vi "Main.vi"(7 "sweep rate, /min":dbl=0.2, 8 "sweep to:":dbl=-0.5, 9 "sweep":T6(radio)=enum."time_sweep") -> ()   [LabVIEW 2017]
uses:
  controls/Channel.ctl
  <instrlib>/Zurich Instruments LabOne/Public/ziTypeHandle.ctl
  controls/Measure.ctl
  controls/iPSreadCtrl.ctl
  controls/iTCreadCtrl.ctl
  subVIs/MFLIcommand.ctl
  controls/iPSsetCtrl.ctl
  controls/Source.ctl
  controls/iTCsetCtrl.ctl
  <vilib>/Utility/file.llb/Write To Spreadsheet File (DBL).vi
  <vilib>/gmath/NI_Gmath.lvlib
  <instrlib>/Keithley 2450/Keithley 2450.lvlib
  HULK SMS/SMScontrols.ctl
  <instrlib>/Zurich Instruments LabOne/Zurich Instruments LabOne.lvlib
panel:
  in  "Lead Chanl":T1(ring)=enum."time_sweep"
  in  "Sweep Up":bool
  in  "Stop Ramp":bool
  in  "Up Rate":dbl
  in  "Down Rate":dbl
  in  "Ramp \nUp":bool
  in  "Ramp\n Down":bool
  in  "lower limit":dbl=-4.0
  in  "upper limit":dbl=4.0
  in  "Sweep Down":bool
  in  "Stop Sweep":bool
  in  "Continuous Sweep":bool
  in  "Slave Chanl":T2=enum."b"
  in  "Double Sweep":bool
  in  "Slope":dbl
  in  "Offset":dbl
  in  "time/point, sec":dbl=2.0
  out "sweep value":dbl=2.186666666666735
  out "time delay, ms":dbl
  out "current time":timestamp=timestamp(3589630313.018 s since 1904-01-01) format="%<%H:%M:%S%1u>T"
  in  "Step and Hyerloop Setups":T3(tab)
  in  "Tab Control":T4(tab)
  in  "MFLI_I2":bool
  in  "MFLI_V2":bool
  in  "MFLI_2":string="DEV5142"
  in  "SR830_8_oop":bool
  in  "SR830_7_oop":bool
  in  "SR830_8_ip":bool
  in  "SR830_7_ip":bool
  in  "SR830_6_oop":bool
  in  "SR830_6_ip":bool
  in  "SR830_8":u8=8
  in  "SR830_7":u8=7
  in  "SR830_6":u8=6
  in  "MFLI_I1":bool
  in  "MFLI_V1":bool
  in  "MFLI_1":string="DEV5150"
  in  "SR830 5 oop":bool
  in  "SR830 5 ip":bool
  in  "SR830 5 addr":u8=5
  in  "SR830 4 oop":bool
  in  "SR830 4 ip":bool
  in  "SR830 3 oop":bool
  in  "SR830 3 ip":bool
  in  "SR830 2 oop":bool
  in  "SR830 2 ip":bool
  in  "SR830 1 oop":bool
  in  "SR830 1 ip":bool
  in  "SR830 4 addr":u8=4
  in  "SR830 3 addr":u8=3
  in  "SR830 2 addr":u8=2
  in  "SR830 1 addr":u8=1
  in  "VTI_P":bool
  in  "PT2_T":bool
  in  "VTI_T":bool
  in  "PT1_T":bool
  in  "SH_T":bool
  in  "Magnet_T":bool
  in  "2182A 4 ch2":bool
  in  "2182A 4 ch1":bool
  in  "2182A 3 ch2":bool
  in  "2182A 3 ch1":bool
  in  "2182A 2 ch2":bool
  in  "2182A 2 ch1":bool
  in  "2182A 4 addr":u8=18
  in  "2182A 3 addr":u8=17
  in  "2182A 2 addr":u8=16
  in  "2182A 1 addr":u8=15
  in  "2182A 1 ch2":bool
  in  "2182A 1 ch1":bool
  out "HandleOut":T5 {"Handle" format="0x%08x"; "Conn" format="0x%08x"}
  out "Handle Out 2":T5 {"Handle" format="0x%08x"; "Conn" format="0x%08x"}
  in  "Step Loop":bool
  in  "Sweep B":bool
  in  "2461_addr_sweep":refnum<visa-resource-name>="itcetherT"
  in  "2461_meas_i":bool
  in  "2461_meas_v":bool
  in  "Tolerance_Sweep":dbl=0.01
  in  "iTC_Sample_T":bool
  in  "iTC_addr_sweep":refnum<visa-resource-name>="iTC"
  in  "iPS_addr_sweep":refnum<visa-resource-name>="iPS"
  in  "2400 3 addr":u8=14
  in  "2400 2 addr":u8=12
  in  "2400 1 addr":u8=13
  in  "2336A addr":refnum<visa-resource-name>="Keithley2614B"
  in  "sweep 2":bool
  in  "iPS_MagnetField":bool
  in  "auto\nrange B":bool
  in  "measure time":bool
  in  "2636A smub meas i":bool
  in  "2636A smub meas v":bool
  in  "2636A smua meas i":bool
  in  "2636A smua meas v":bool
  in  "2400 3 meas i":bool
  in  "2400 2 meas i":bool
  in  "2400 2 meas v":bool
  in  "2400 3 meas v":bool
  in  "2400 1 meas i":bool
  in  "2400 1 meas v":bool
  in  "auto\nrange A":bool
  in  "SlaveUpLimit":dbl
  in  "SlaveDownLimit":dbl
  in  "Change Doule Sweep OffSet":bool
  in  "Lead Chanl_step":T7(ring)=enum."2636a_smua_step" caption="Lead Chanl"
  in  "UpLimitValue":dbl
  in  "DownLimitValue":dbl
  in  "Change Sweep Range":bool
  in  "Offset_Up":dbl
  in  "Offset_Down":dbl
  in  "Slope":dbl
  in  "Down          Up":string[][](table)
  in  "Generate":bool
  in  "2461_addr_step":refnum<visa-resource-name>="itcetherT"
  in  "Channel":T2=enum."b"
  in  "Mini steps":dbl=30.0
  in  "Tolerance_Step":dbl=0.01
  in  "Step Slope":dbl
  in  "Step Offset":dbl
  in  "diagonal step":bool
  in  "FieldRate(T/min)":dbl=0.1
  out "at field":bool
  in  "iPS _addr_step":refnum<visa-resource-name>="iPS"
  in  "iTC_addr_step":refnum<visa-resource-name>="iTC"
  in  "step":T8(radio)=enum."time_step"
  in  "2336A_addr_step":refnum<visa-resource-name>="Keithley2614B"
  in  "2400_2_addr_step":u8=12
  in  "2400_1_addr_step":u8=12
  in  "wait between sweeps(s)":u32=1
  in  "Wait Between Step(s)":i32=1
  in  "Stop Mapping":bool
  in  "Start Mapping":bool
  in  "HyperLoop":bool
  in  "EstimateTime":bool
  out "MM:":dbl
  out "SS:":dbl
  out "HH:":dbl
  out "Finish Time":timestamp
  out "Sweep Direction":string
  out "Current Step Value":dbl
  out "Table Index":dbl
  in  "Populate step table?":bool
  in  "Step values":string[][](table)=[["-20"], ["-10"], ["-4"], ["-1"], ["3"], ["6"], ["10"], [""]]
  in  "to":dbl=1.0
  in  "step":dbl=2.0
  in  "from":dbl=1.0
  in  "SwapStepDirection":bool
  out "Hidden_HyperLoop_Swap":bool
  out "HyperLoop Hidden":bool
  in  "EstimateTime Hyper":bool
  out "MM:":dbl
  out "SS:":dbl
  out "HH:":dbl
  out "Finish Time 2":timestamp
  out "Sweep Direction 2":string
  out "Current Hyper Value":dbl
  out "HyperLoop Index":dbl
  in  "Populate HyperLoop table?":bool
  in  "HyperLoop Steps":string[][](table)=[["-20"], ["-10"], ["-4"], ["-1"], ["3"], ["6"], ["10"], [""]]
  in  "to":dbl=1.0
  in  "step":dbl=2.0
  in  "from":dbl=1.0
  in  "SuperHyper":bool
  in  "Channel_hyper":T2=enum."b"
  in  "Hyper_Mini steps":dbl=30.0
  in  "Tolerance_Hyper":dbl=0.1
  in  "Hyper Slope":dbl
  in  "Hyper Offset":dbl
  in  "diagonal_hyper":bool
  in  "Hyper_FieldRate\n(T/min)":dbl=0.1
  out "at field_hyper":bool
  in  "iPS _addr_hyper":refnum<visa-resource-name>="iPS"
  in  "iTC_addr_hyper":refnum<visa-resource-name>="iTC"
  in  "step_hyper":T9(radio)=enum."time_HyperLoop"
  in  "2336A_addr_hyper":refnum<visa-resource-name>="Keithley2614B"
  in  "2400_2_addr_hyper":u8=12
  in  "2400_1_addr_hyper":u8=12
  in  "Wait Between Hyper":i32=10
  in  "Stop HyperLoop":bool
  in  "Start HyperLoop":bool
  in  "SwapHyperDirection":bool
  out "Hidden_super_Swap":bool
  out "Super Hidden":bool
  in  "EstimateTime Hyper 2":bool
  out "MM:":dbl
  out "SS:":dbl
  out "HH:":dbl
  out "Finish Time Super":timestamp
  out "Sweep Direction3":string
  out "Current SuperHyper Value":dbl
  out "SuperHyper_Index":dbl
  in  "Populate SuperHyper table?":bool
  in  "SuperHyper Steps":string[][](table)=[["-20"], ["-10"], ["-4"], ["-1"], ["3"], ["6"], ["10"], [""]]
  in  "to":dbl=1.0
  in  "step":dbl=2.0
  in  "from":dbl=1.0
  in  "Channel_super":T2=enum."b"
  in  "Super_ministeps":dbl=30.0
  in  "Tolerance_super":dbl=0.1
  in  "Slope_super":dbl
  in  "Offset_super":dbl
  in  "diagona_super":bool
  in  "Super_FieldRate\n(T/min)":dbl=0.1
  out "at field_super":bool
  in  "iPS _addr_superhyper":refnum<visa-resource-name>="iPS"
  in  "iTC_addr_super":refnum<visa-resource-name>="iTC"
  in  "step_super":T10(radio)=enum."time_SuperHyper"
  in  "2336A_addr_super":refnum<visa-resource-name>="Keithley2614B"
  in  "2400_2_addr_super":u8=12
  in  "2400_1_addr_super":u8=12
  in  "Wait Btwn SuperHyper":i32=10
  in  "Stop SuperHyper":bool
  in  "StartSuperHyper":bool
  out "SuperHyper":dbl=-0.4901
  out "Hyper Channel":dbl=-0.4901
  out "Sweep Channel":dbl
  out "Step Channel":dbl=-0.4901
  in  "MappingName":string
  in  "Data Folder":path=path "F:/users/Yanmeng/Data"
  out "Data file:":path=path "D:/Yanmeng/Data/Year2018/January2018/Jan2318/Jan2318x001.dat"
  in  "Initialize":bool
  in  "Quit":bool
  in  "Refresh Time(ms)":u32=100
  in  "Monitor":bool
  out "DownNameString":string
  out "UpNameString":string
  in  "Cytec_Switch":bool
  in  "Lockin_Setup":bool
  in  "TempCtrl":bool
  in  "MagnetCtrl":bool
  out "status 3":bool
  in  "Y_right_formula":string="brty/10/(300*10^-9)"
  in  "Yright":u16(ring)=3 caption="Y-Right:" items=["V_sweep_2636a_smub", "SR830_1_ip", "SR830_1_oop", "SR830_2_ip", "SR830_2_oop", "SR830_3_ip", "SR830_3_oop", "SR830_4_ip", "SR830_4_oop", "2636A_smua_v", "2636A_smua_i", "2636A_smub_v", "2636A_smub_i", "iPS_MagntField", "iPS_Magnet_T", "iPS_SH_T", "iTC_Sample_T", "iTC_VTI_T", "iTC_PT1_T", "iTC_PT2_T", "iTC_VTI_P", "formula"]
  out "status 2":bool
  in  "Y_left_formula":string="brty/10/(300*10^-9)"
  in  "X_axis_formula":string
  in  "Yaxis":u16(ring)=3 caption="Y-Left:" items=["V_sweep_2636a_smub", "SR830_1_ip", "SR830_1_oop", "SR830_2_ip", "SR830_2_oop", "SR830_3_ip", "SR830_3_oop", "SR830_4_ip", "SR830_4_oop", "2636A_smua_v", "2636A_smua_i", "2636A_smub_v", "2636A_smub_i", "iPS_MagntField", "iPS_Magnet_T", "iPS_SH_T", "iTC_Sample_T", "iTC_VTI_T", "iTC_PT1_T", "iTC_PT2_T", "iTC_VTI_P", "formula"]
  out "XY Graph":cluster{"Y Values":dbl[], "Y Values":dbl[]}[](graph)
  in  "Xaxis":u16(ring) caption="X-axis:" items=["V_sweep_2636a_smub", "SR830_1_ip", "SR830_1_oop", "SR830_2_ip", "SR830_2_oop", "SR830_3_ip", "SR830_3_oop", "SR830_4_ip", "SR830_4_oop", "2636A_smua_v", "2636A_smua_i", "2636A_smub_v", "2636A_smub_i", "iPS_MagntField", "iPS_Magnet_T", "iPS_SH_T", "iTC_Sample_T", "iTC_VTI_T", "iTC_PT1_T", "iTC_PT2_T", "iTC_VTI_P", "formula"]
  out "status":bool
  in  "Show cursor":bool
  in  "Hulk_B_meas (Vnano)":bool
  in  "Hulk_SMS_addr":refnum<visa-resource-name>="TCPIP0::10.99.75.17::inst0::INSTR"
  in  "formula_variables":string[](array[string])=["a", "b", "c", "d", "e", "e", "f", "g", "h", "i", "j"]
  out "data":dbl[](array[numeric])
  out "Figure_axis":string[](array[string])=["HULK_SMS_output", "SR830_1_ip", "SR830_1_oop"]
  out "data_caption":string="HULK_SMS_output\tSR830_1_ip\tSR830_1_oop\t"
  # "Sweep Parameters Setup"
  # "Down"
  # "Up"
  # "Limits"
  # "Rate\n(/min)"
  # "Sweep Channel Setup"
  # "SweepChannel"
  # "address"
  # "sweep"
  # "2400_2"
  # "2400_3"
  # "2636A_smua"
  # "2636A_smub"
  # "time"
  # "Teslatron iPS"
  # "Teslatron iTC"
  # "2400_1"
  # "!Current sweep!"
  # "measure"
  # "Sample_T"
  # "MagnetField"
  # "voltage (_v)"
  # "current (_i)"
  # "Vtg"
  # "Vbg"
  # "Measure Channels"
  # "Lock-in amplifiers"
  # "address"
  # "SR830_1"
  # "SR830_2"
  # "SR830_3"
  # "SR830_4"
  # "measure"
  # "SR830_5"
  # "in phase (_ip)"
  # "out of phase (_oop)"
  # "Nanovoltmeters"
  # "Magnet&Temp"
  # "address"
  # "Equipment"
  # "iPS"
  # "iTC"
  # "measure"
  # "2182A_1"
  # "2182A_2"
  # "2182A_3"
  # "2182A_4"
  # "channel 1 (_ch1)"
  # "channel 2 (_ch2)"
  # "(not recommended, slow)"
  # "Step Channel Setup"
  # "StepChannel"
  # "addres"
  # "time"
  # "2400_1"
  # "2400_2"
  # "2636A_smua"
  # "2636A_smub"
  # "Teslatron iPS"
  # "Teslatron iTC"
  # "2461"
  # "step"
  # "Step Table"
  # "Step Table"
  # "Hyper Loop Setup"
  # "StepChannel"
  # "addres"
  # "Teslatron iPS"
  # "Teslatron iTC"
  # "2400_1"
  # "2400_2"
  # "2636A_smua"
  # "2636A_smub"
  # "time"
  # "step"
  # "SuperHyper Setup"
  # "StepChannel"
  # "addres"
  # "2400_1"
  # "2400_2"
  # "2636A_smua"
  # "2636A_smub"
  # "time"
  # "Teslatron iPS"
  # "Teslatron iTC"
  # "step"
  # "Step Table"
  # "Current Value of Sweep and Step Channels"
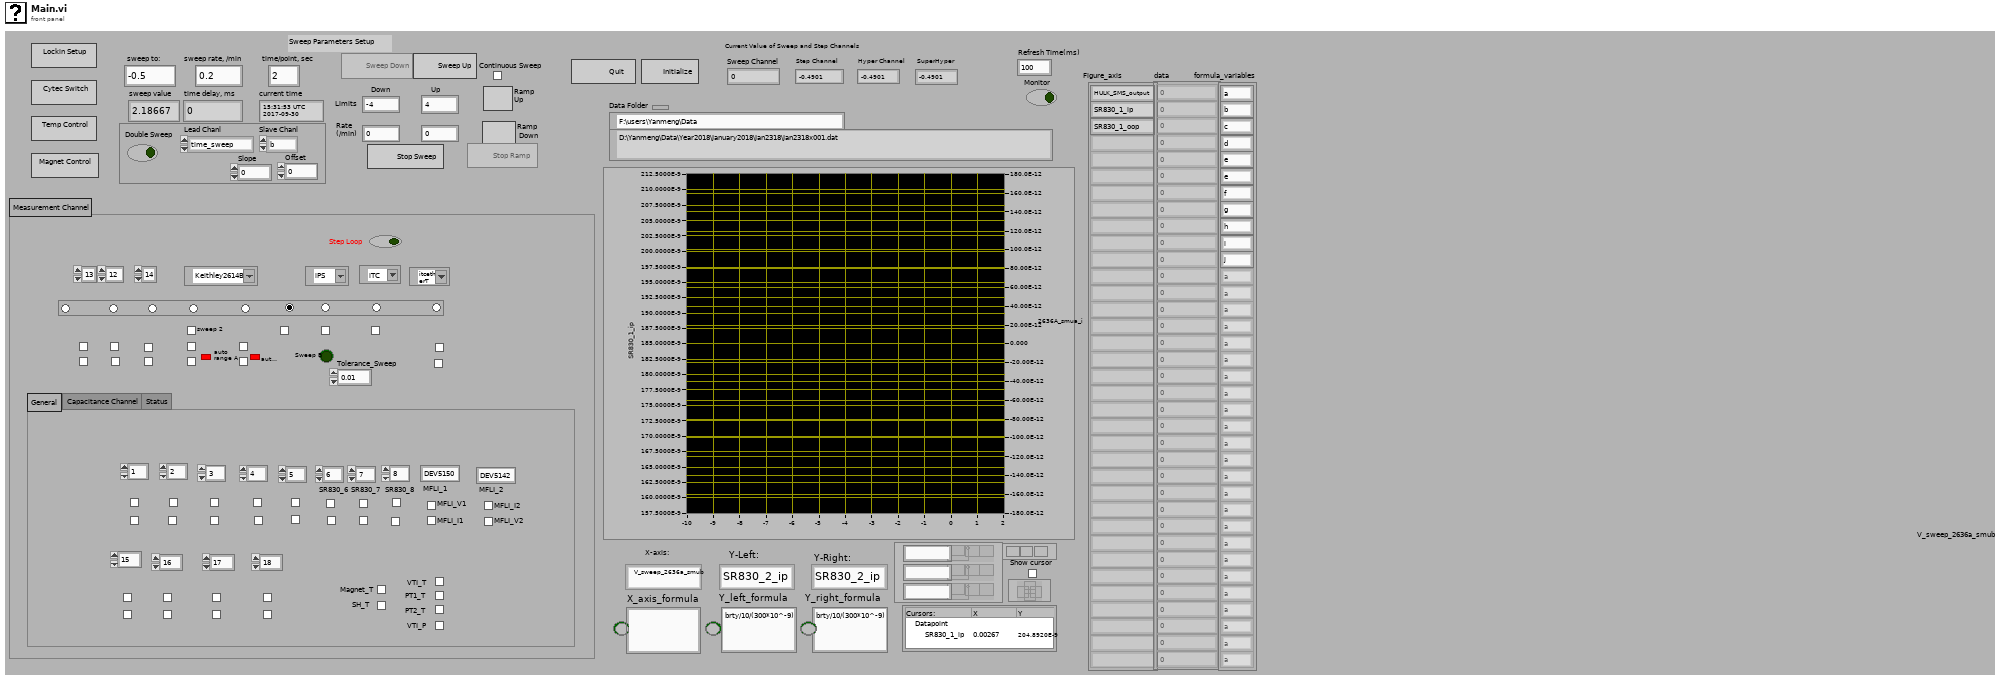
[diagram p1: front panel]
types:
  T1 = enum16{"2400_1", "2400_2", "2400_3", "2636a_smua", "2636a_smub", "time_sweep", "iPS", "iTC", "2461"}
  T2 = typedef "Channel.ctl" = enum16{"a", "b"}
  T3 = enum32{"Measurement Channel", "Step", "HyperLoop", "SuperHyper"}
  T4 = enum32{"General", "Capacitance Channel", "Status"}
  T5 = typedef "Zurich Instruments LabOne.lvlib/ziTypeHandle.ctl" = cluster{"handleValid":bool, "Conn":u64, "Path Prefix":string, "Handle":u64, "Connected":bool, "Clockbase(s)":dbl}
  T6 = enum32{"2400_1", "2400_2", "2400_3", "2636a_smua", "2636a_smub", "time_sweep", "iPS", "iTC", "2461"}
  T7 = enum16{"V2400_1_step", "V2400_2_step", "2636a_smua_step", "2636a_smub_step", "time_step", "iPS_step", "iTC_step", "2461_Curr"}
  T8 = enum32{"V2400_1_Step", "V2400_2_step", "2636_smua_step", "2636_smub_step", "time_step", "iTC_step", "iPS_step", "2461_Curr"}
  T9 = enum32{"2400_1_HyperLoop", "2400_2_HyperLoop", "2636_smua_HyperLoop", "2636_smub_HyperLoop", "time_HyperLoop", "iTC_HyperLoop", "iPS_HyperLoop"}
  T10 = enum32{"2400_1_SuperHyper", "2400_2_SuperHyper", "2636_smua_SuperHyper", "2636_smub_SuperHyper", "time_SuperHyper", "iTC_SuperHyper", "iPS_SuperHyper"}
  T11 = cluster{"vi reference":refnum<vi>, "vi reference":refnum<vi>}
  T12 = enum8{"Enabled", "Disabled", "Disabled and Grayed Out"}
  T13 = typedef "Measure.ctl" = enum16{"Voltage", "Current", "Resistance", "Power"}
  T14 = typedef "SMScontrols.ctl" = enum16{"UPDATE", "GET OUTPUT", "RAMP ZERO", "RAMP MID", "RAMP MAX", "RAMP STATUS", "PAUSE OFF", "PAUSE ON", "HEATER OFF", "HEATER ON", "TESLA OFF", "TESLA ON", "DIRECTION +", "DIRECTION -", "DIRECTION 0", "SET MID", "SET MAX", "SET RAMP", "SET LIMIT", "SET TPA", "SET HEATER"}
  T15 = typedef "iPSreadCtrl.ctl" = enum16{"OutputField", "MagnetField", "Switch Heater Temp", "Field Rate", "Magnet Temp", "OutputVoltage"}
  T16 = typedef "iTCreadCtrl.ctl" = enum16{"PT1 Temp", "PT2 Temp", "Sample Temp", "VTI Temp", "Needle Valve", "VTI Heater Power", "Sample Heater Power", "VTI Pressure"}
  T17 = typedef "MFLIcommand.ctl" = enum16{"initialyze", "measure current", "measure XY on demod0", "Set AuxOut1", "Set AuxOut2", "Set AuxOut3", "Set AuxOut4", "Set Osc Ampl", "SigIns Autorange", "finalyze", "Set Osc1 Freq"}
  T18 = typedef "iPSsetCtrl.ctl" = enum16{"Set Target Field", "Set Target Field Rate", "Switch Heater ON", "Switch Heater OFF", "Go to Field", "Go to Zero", "Hold"}
  T19 = enum32{"Radio Selection 1", "Radio Selection 2", "Radio Selection 3", "Radio Selection 4", "Radio Selection 5", "Radio Selection 6", "Radio Selection 7"}
  T20 = typedef "Source.ctl" = enum16{"Current", "Voltage"}
  T21 = typedef "iTCsetCtrl.ctl" = enum16{"Set Sample Temp", "Set VTI Temp", "Set Needle Valve", "Set VTI Heater Power", "Set Sample Heater Power", "Set VTI Pressure"}
  T22 = typedef "Zurich Instruments LabOne.lvlib/ziTypeDemodSampleSingle.ctl" = cluster{"Timestamps (ticks)":u64, "X (Vrms)":dbl, "Y (Vrms)":dbl, "Osc Phase (deg)":dbl, "Freq (Hz)":dbl, "DIO":u32, "AuxIn0 (V)":dbl, "AuxIn1 (V)":dbl, "Trigger":u32}
  T23 = enum32{"Bad", "Idle", "Run top level", "Running"}
diagram:
  # "This template is for the Producer/Consumer design pattern."
  # "initial value"
  n1 = flat-sequence {
    tunnel: [w15] -> w2
    tunnel: [w7] -> w1
    frame #0 {
      n2 = Current VI's Path() -> (path=w22:path)
      n3 = Strip Path(path=w22) -> (stripped path=w13:path)  [unwired: 1 out]
      n4 = Build Path(base path=w13, name or relative path="subVIs\\MagnetControl.vi") -> (appended path=w18:path)
      n5 = Build Path(base path=w13, name or relative path="subVIs\\TemperatureControl.vi") -> (appended path=w19:path)
      n6 = Build Path(base path=w13, name or relative path="subVIs\\CytecControl.vi") -> (appended path=w11:path)
      n7 = Build Path(base path=w13, name or relative path="subVIs\\Lockin Control Panel.vi") -> (appended path=w10:path)
      n8 = Open VI Reference(vi path=w18) -> (vi reference=w16:refnum<vi>)  [unwired: 5 in, 1 out]
      n9 = Open VI Reference(vi path=w19) -> (vi reference=w17:refnum<vi>)  [unwired: 5 in, 1 out]
      n10 = Open VI Reference(vi path=w10) -> (vi reference=w8:refnum<vi>)  [unwired: 5 in, 1 out]
      n11 = Open VI Reference(vi path=w11) -> (vi reference=w9:refnum<vi>)  [unwired: 5 in, 1 out]
      n12 = Bundle("vi reference"=w9, "vi reference"=w8) -> (w7:T11)  [unwired: 1 in]
      n13 = Bundle("vi reference"=w17, "vi reference"=w16) -> (w15:T11)  [unwired: 1 in]
    }
    frame #1 {
      w24 = T12."Disabled and Grayed Out" ("Disabled")
      w26 = T12."Enabled" ("Disabled")
      # "1 = 2400 1\n2 = 2400 2\n3 = 2400 3\n4 = 2636a smua\n5 = 2636a smub\n6 = do not sweep, just time\n7 = Magnetic Field IPS120\n8= 2461 smu"
      # "delete previous values"
      n14 = property on="Step Loop" class="Bool (strict)"() -> ("Value"=w25:bool)  [unwired: 2 in, 2 out]
      n15 = case shown="True" w25 {
        frame False {
          w29 = FALSE ("Change Sweep Range")
          w35 = FALSE ("Visible")
          w30 = FALSE ("HyperLoop")
          w36 = T12."Disabled and Grayed Out" ("Disabled")
          w42 = T12."Enabled" ("Disabled")
          n16 = property on="UpLimitValue" class="DigNum (strict)"("Visible"=w35) -> ()  [unwired: 2 in, 2 out]
          n17 = property on="DownLimitValue" class="DigNum (strict)"("Visible"=w35) -> ()  [unwired: 2 in, 2 out]
          n18 = property on="Generate" class="Bool"("Visible"=w35) -> ()  [unwired: 2 in, 2 out]
          n19 = property on="Offset_Up" class="DigNum (strict)"("Visible"=w35) -> ()  [unwired: 2 in, 2 out]
          n20 = property on="Down          Up" class="Tbl (strict)"("Visible"=w35) -> ()  [unwired: 2 in, 2 out]
          n21 = property on="Slope" class="DigNum (strict)"("Visible"=w35) -> ()  [unwired: 2 in, 2 out]
          n22 = property on="Offset_Down" class="DigNum (strict)"("Visible"=w35) -> ()  [unwired: 2 in, 2 out]
          n23 = property on="Change Sweep Range" class="Bool (strict)"("Value"=w29) -> ()  [unwired: 2 in, 2 out]
          n24 = property on="SwapHyperDirection" class="Bool (strict)"("Value"=w29) -> ()  [unwired: 2 in, 2 out]
          n25 = property on="Tolerance_Sweep" class="DigNum (strict)"("DisabledEnum"=w42) -> ()  [unwired: 2 in, 2 out]
          n26 = property on="Ramp\n Down" class="Bool"("DisabledEnum"=w42) -> ()  [unwired: 2 in, 2 out]
          n27 = property on="sweep" class="RadioBtnsControl (strict)"("DisabledEnum"=w42) -> ()  [unwired: 2 in, 2 out]
          n28 = property on="2182A 1 addr" class="DigNum (strict)"("DisabledEnum"=w42) -> ()  [unwired: 2 in, 2 out]
          n29 = property on="2182A 2 addr" class="DigNum (strict)"("DisabledEnum"=w42) -> ()  [unwired: 2 in, 2 out]
          n30 = property on="2182A 3 addr" class="DigNum (strict)"("DisabledEnum"=w42) -> ()  [unwired: 2 in, 2 out]
          n31 = property on="2182A 4 addr" class="DigNum (strict)"("DisabledEnum"=w42) -> ()  [unwired: 2 in, 2 out]
          n32 = property on="2400 1 addr" class="DigNum (strict)"("DisabledEnum"=w42) -> ()  [unwired: 2 in, 2 out]
          n33 = property on="Continuous Sweep" class="Bool (strict)"("DisabledEnum"=w42) -> ()  [unwired: 2 in, 2 out]
          n34 = property on="Sweep Down" class="Bool"("DisabledEnum"=w42) -> ()  [unwired: 2 in, 2 out]
          n35 = property on="Sweep Up" class="Bool"("DisabledEnum"=w42) -> ()  [unwired: 2 in, 2 out]
          n36 = property on="SR830 2 addr" class="DigNum (strict)"("DisabledEnum"=w42) -> ()  [unwired: 2 in, 2 out]
          n37 = property on="SR830 3 addr" class="DigNum (strict)"("DisabledEnum"=w42) -> ()  [unwired: 2 in, 2 out]
          n38 = property on="2400 2 addr" class="DigNum (strict)"("DisabledEnum"=w42) -> ()  [unwired: 2 in, 2 out]
          n39 = property on="2400 3 addr" class="DigNum (strict)"("DisabledEnum"=w42) -> ()  [unwired: 2 in, 2 out]
          n40 = property on="2336A addr" class="VISAName"("DisabledEnum"=w42) -> ()  [unwired: 2 in, 2 out]
          n41 = property on="SR830 1 addr" class="DigNum (strict)"("DisabledEnum"=w42) -> ()  [unwired: 2 in, 2 out]
          n42 = property on="SR830 4 addr" class="DigNum (strict)"("DisabledEnum"=w42) -> ()  [unwired: 2 in, 2 out]
          n43 = property on="Ramp \nUp" class="Bool"("DisabledEnum"=w42) -> ()  [unwired: 2 in, 2 out]
          n44 = property on="Step and Hyerloop Setups" class="TabCtl (strict)"() -> ("Pages"=w31:refnum<vi>[])  [unwired: 2 in, 2 out]
          n45 = property on="Step and Hyerloop Setups" class="TabCtl (strict)"() -> ("Pages"=w40:refnum<vi>[])  [unwired: 2 in, 2 out]
          n46 = Index Array(array=w31, index=2) -> (element=w32:refnum<vi>)
          n47 = Index Array(array=w40, index=1) -> (element=w39:refnum<vi>)
          n48 = property class="Page"(reference=w32, "PageVis"=FALSE ("Page Visible")) -> ()  [unwired: 1 in, 2 out]
          n49 = property class="Page"(reference=w39, "PageVis"=FALSE ("Page Visible")) -> ()  [unwired: 1 in, 2 out]
          n50 = property on="HyperLoop" class="Bool (strict)"("Value"=w30) -> ()  [unwired: 2 in, 2 out]
          n51 = property on="SuperHyper" class="Bool (strict)"("Value"=w30) -> ()  [unwired: 2 in, 2 out]
          n52 = property on="MappingName" class="Str"("Visible"=FALSE) -> ()  [unwired: 2 in, 2 out]
          n53 = property on="step" class="RadioBtnsControl (strict)"("DisabledEnum"=w36) -> ()  [unwired: 2 in, 2 out]
          n54 = property on="diagonal step" class="Bool (strict)"("DisabledEnum"=w36) -> ()  [unwired: 2 in, 2 out]
          n55 = property on="FieldRate(T/min)" class="DigNum (strict)"("DisabledEnum"=w36) -> ()  [unwired: 2 in, 2 out]
          n56 = property on="Step Offset" class="DigNum (strict)"("DisabledEnum"=w36) -> ()  [unwired: 2 in, 2 out]
          n57 = property on="Tolerance_Step" class="DigNum (strict)"("DisabledEnum"=w36) -> ()  [unwired: 2 in, 2 out]
          n58 = property on="Step Slope" class="DigNum (strict)"("DisabledEnum"=w36) -> ()  [unwired: 2 in, 2 out]
          n59 = property on="iPS _addr_step" class="VISAName"("DisabledEnum"=w36) -> ()  [unwired: 2 in, 2 out]
          n60 = property on="wait between sweeps(s)" class="DigNum (strict)"("DisabledEnum"=w36) -> ()  [unwired: 2 in, 2 out]
          n61 = property on="2336A_addr_step" class="VISAName"("DisabledEnum"=w36) -> ()  [unwired: 2 in, 2 out]
          n62 = property on="iTC_addr_step" class="VISAName"("DisabledEnum"=w36) -> ()  [unwired: 2 in, 2 out]
          n63 = property on="Start Mapping" class="Bool"("DisabledEnum"=w36) -> ()  [unwired: 2 in, 2 out]
          n64 = property on="2400_1_addr_step" class="DigNum (strict)"("DisabledEnum"=w36) -> ()  [unwired: 2 in, 2 out]
          n65 = property on="Wait Between Step(s)" class="DigNum (strict)"("DisabledEnum"=w36) -> ()  [unwired: 2 in, 2 out]
          n66 = property on="2400_2_addr_step" class="DigNum (strict)"("DisabledEnum"=w36) -> ()  [unwired: 2 in, 2 out]
          n67 = property on="HyperLoop" class="Bool (strict)"("DisabledEnum"=w36) -> ()  [unwired: 2 in, 2 out]
        }
        frame True {
          w47 = FALSE ("Change Sweep Range")
          w53 = FALSE ("Visible")
          w48 = FALSE ("HyperLoop")
          w60 = T12."Disabled and Grayed Out" ("Disabled")
          w54 = T12."Enabled" ("Disabled")
          n68 = property on="UpLimitValue" class="DigNum (strict)"("Visible"=w53) -> ()  [unwired: 2 in, 2 out]
          n69 = property on="DownLimitValue" class="DigNum (strict)"("Visible"=w53) -> ()  [unwired: 2 in, 2 out]
          n70 = property on="Generate" class="Bool"("Visible"=w53) -> ()  [unwired: 2 in, 2 out]
          n71 = property on="Offset_Up" class="DigNum (strict)"("Visible"=w53) -> ()  [unwired: 2 in, 2 out]
          n72 = property on="Down          Up" class="Tbl (strict)"("Visible"=w53) -> ()  [unwired: 2 in, 2 out]
          n73 = property on="Slope" class="DigNum (strict)"("Visible"=w53) -> ()  [unwired: 2 in, 2 out]
          n74 = property on="Offset_Down" class="DigNum (strict)"("Visible"=w53) -> ()  [unwired: 2 in, 2 out]
          n75 = property on="SwapHyperDirection" class="Bool (strict)"("Value"=w47) -> ()  [unwired: 2 in, 2 out]
          n76 = property on="Change Sweep Range" class="Bool (strict)"("Value"=w47) -> ()  [unwired: 2 in, 2 out]
          n77 = property on="Ramp\n Down" class="Bool"("DisabledEnum"=w60) -> ()  [unwired: 2 in, 2 out]
          n78 = property on="sweep" class="RadioBtnsControl (strict)"("DisabledEnum"=w60) -> ()  [unwired: 2 in, 2 out]
          n79 = property on="2182A 1 addr" class="DigNum (strict)"("DisabledEnum"=w60) -> ()  [unwired: 2 in, 2 out]
          n80 = property on="2182A 2 addr" class="DigNum (strict)"("DisabledEnum"=w60) -> ()  [unwired: 2 in, 2 out]
          n81 = property on="2182A 3 addr" class="DigNum (strict)"("DisabledEnum"=w60) -> ()  [unwired: 2 in, 2 out]
          n82 = property on="2182A 4 addr" class="DigNum (strict)"("DisabledEnum"=w60) -> ()  [unwired: 2 in, 2 out]
          n83 = property on="2400 1 addr" class="DigNum (strict)"("DisabledEnum"=w60) -> ()  [unwired: 2 in, 2 out]
          n84 = property on="Tolerance_Sweep" class="DigNum (strict)"("DisabledEnum"=w60) -> ()  [unwired: 2 in, 2 out]
          n85 = property on="Sweep Down" class="Bool"("DisabledEnum"=w60) -> ()  [unwired: 2 in, 2 out]
          n86 = property on="SR830 2 addr" class="DigNum (strict)"("DisabledEnum"=w60) -> ()  [unwired: 2 in, 2 out]
          n87 = property on="SR830 3 addr" class="DigNum (strict)"("DisabledEnum"=w60) -> ()  [unwired: 2 in, 2 out]
          n88 = property on="2400 2 addr" class="DigNum (strict)"("DisabledEnum"=w60) -> ()  [unwired: 2 in, 2 out]
          n89 = property on="2400 3 addr" class="DigNum (strict)"("DisabledEnum"=w60) -> ()  [unwired: 2 in, 2 out]
          n90 = property on="2336A addr" class="VISAName"("DisabledEnum"=w60) -> ()  [unwired: 2 in, 2 out]
          n91 = property on="SR830 1 addr" class="DigNum (strict)"("DisabledEnum"=w60) -> ()  [unwired: 2 in, 2 out]
          n92 = property on="SR830 4 addr" class="DigNum (strict)"("DisabledEnum"=w60) -> ()  [unwired: 2 in, 2 out]
          n93 = property on="Ramp \nUp" class="Bool"("DisabledEnum"=w60) -> ()  [unwired: 2 in, 2 out]
          n94 = property on="Step and Hyerloop Setups" class="TabCtl (strict)"() -> ("Pages"=w49:refnum<vi>[])  [unwired: 2 in, 2 out]
          n95 = property on="Step and Hyerloop Setups" class="TabCtl (strict)"() -> ("Pages"=w46:refnum<vi>[])  [unwired: 2 in, 2 out]
          n96 = property on="Step and Hyerloop Setups" class="TabCtl (strict)"() -> ("Pages"=w58:refnum<vi>[])  [unwired: 2 in, 2 out]
          n97 = property on="Continuous Sweep" class="Bool (strict)"("DisabledEnum"=w60) -> ()  [unwired: 2 in, 2 out]
          n98 = property on="Continuous Sweep" class="Bool (strict)"("Value"=FALSE ("Continuous Sweep")) -> ()  [unwired: 2 in, 2 out]
          n99 = Index Array(array=w49, index=2) -> (element=w50:refnum<vi>)
          n100 = Index Array(array=w46, index=3) -> (element=w45:refnum<vi>)
          n101 = Index Array(array=w58, index=1) -> (element=w57:refnum<vi>)
          n102 = property on="SuperHyper" class="Bool (strict)"("Value"=w48) -> ()  [unwired: 2 in, 2 out]
          n103 = property on="HyperLoop" class="Bool (strict)"("Value"=w48) -> ()  [unwired: 2 in, 2 out]
          n104 = property class="Page"(reference=w50, "PageVis"=FALSE ("Page Visible")) -> ()  [unwired: 1 in, 2 out]
          n105 = property class="Page"(reference=w45, "PageVis"=FALSE ("Page Visible")) -> ()  [unwired: 1 in, 2 out]
          n106 = property on="MappingName" class="Str"("Visible"=TRUE) -> ()  [unwired: 2 in, 2 out]
          n107 = property class="Page"(reference=w57, "PageVis"=FALSE ("Page Visible")) -> ()  [unwired: 1 in, 2 out]
          n108 = property on="step" class="RadioBtnsControl (strict)"("DisabledEnum"=w54) -> ()  [unwired: 2 in, 2 out]
          n109 = property on="Step Offset" class="DigNum (strict)"("DisabledEnum"=w54) -> ()  [unwired: 2 in, 2 out]
          n110 = property on="diagonal step" class="Bool (strict)"("DisabledEnum"=w54) -> ()  [unwired: 2 in, 2 out]
          n111 = property on="Step Slope" class="DigNum (strict)"("DisabledEnum"=w54) -> ()  [unwired: 2 in, 2 out]
          n112 = property on="iPS _addr_step" class="VISAName"("DisabledEnum"=w54) -> ()  [unwired: 2 in, 2 out]
          n113 = property on="wait between sweeps(s)" class="DigNum (strict)"("DisabledEnum"=w54) -> ()  [unwired: 2 in, 2 out]
          n114 = property on="FieldRate(T/min)" class="DigNum (strict)"("DisabledEnum"=w54) -> ()  [unwired: 2 in, 2 out]
          n115 = property on="2336A_addr_step" class="VISAName"("DisabledEnum"=w54) -> ()  [unwired: 2 in, 2 out]
          n116 = property on="iTC_addr_step" class="VISAName"("DisabledEnum"=w54) -> ()  [unwired: 2 in, 2 out]
          n117 = property on="Start Mapping" class="Bool"("DisabledEnum"=w54) -> ()  [unwired: 2 in, 2 out]
          n118 = property on="2400_1_addr_step" class="DigNum (strict)"("DisabledEnum"=w54) -> ()  [unwired: 2 in, 2 out]
          n119 = property on="Wait Between Step(s)" class="DigNum (strict)"("DisabledEnum"=w54) -> ()  [unwired: 2 in, 2 out]
          n120 = property on="Tolerance_Step" class="DigNum (strict)"("DisabledEnum"=w54) -> ()  [unwired: 2 in, 2 out]
          n121 = property on="2400_2_addr_step" class="DigNum (strict)"("DisabledEnum"=w54) -> ()  [unwired: 2 in, 2 out]
          n122 = property on="HyperLoop" class="Bool (strict)"("DisabledEnum"=w54) -> ()  [unwired: 2 in, 2 out]
        }
      }
      n123 = property on="time delay, ms" class="DigNum (strict)"("Value"=u32 0 ("delib time delay")) -> ()  [unwired: 2 in, 2 out]
      n124 = local write "data"(dbl[] [] ("data")) -> ()
      n125 = property on="Monitor" class="Bool (strict)"() -> ("Value"=w23:bool)  [unwired: 2 in, 2 out]
      n126 = property on="formula_variables" class="Arr (strict)"("Visible"=w23) -> ()  [unwired: 2 in, 2 out]
      n127 = property on="data" class="Arr (strict)"("Visible"=w23) -> ()  [unwired: 2 in, 2 out]
      n128 = property on="Figure_axis" class="Arr (strict)"("Visible"=w23) -> ()  [unwired: 2 in, 2 out]
      n129 = property on="Stop Mapping" class="Bool"("DisabledEnum"=w24) -> ()  [unwired: 2 in, 2 out]
      n130 = property on="Stop Sweep" class="Bool"("DisabledEnum"=w24) -> ()  [unwired: 2 in, 2 out]
      n131 = property on="Stop Ramp" class="Bool"("DisabledEnum"=w24) -> ()  [unwired: 2 in, 2 out]
      n132 = property on="sweep" class="RadioBtnsControl (strict)"("DisabledEnum"=w26) -> ()  [unwired: 2 in, 2 out]
      n133 = property on="2182A 1 addr" class="DigNum (strict)"("DisabledEnum"=w26) -> ()  [unwired: 2 in, 2 out]
      n134 = property on="2182A 2 addr" class="DigNum (strict)"("DisabledEnum"=w26) -> ()  [unwired: 2 in, 2 out]
      n135 = property on="2182A 3 addr" class="DigNum (strict)"("DisabledEnum"=w26) -> ()  [unwired: 2 in, 2 out]
      n136 = property on="2182A 4 addr" class="DigNum (strict)"("DisabledEnum"=w26) -> ()  [unwired: 2 in, 2 out]
      n137 = property on="2400 1 addr" class="DigNum (strict)"("DisabledEnum"=w26) -> ()  [unwired: 2 in, 2 out]
      n138 = property on="SR830 2 addr" class="DigNum (strict)"("DisabledEnum"=w26) -> ()  [unwired: 2 in, 2 out]
      n139 = property on="SR830 3 addr" class="DigNum (strict)"("DisabledEnum"=w26) -> ()  [unwired: 2 in, 2 out]
      n140 = property on="2400 2 addr" class="DigNum (strict)"("DisabledEnum"=w26) -> ()  [unwired: 2 in, 2 out]
      n141 = property on="2400 3 addr" class="DigNum (strict)"("DisabledEnum"=w26) -> ()  [unwired: 2 in, 2 out]
      n142 = property on="2336A addr" class="VISAName"("DisabledEnum"=w26) -> ()  [unwired: 2 in, 2 out]
      n143 = property on="SR830 1 addr" class="DigNum (strict)"("DisabledEnum"=w26) -> ()  [unwired: 2 in, 2 out]
      n144 = property on="SR830 4 addr" class="DigNum (strict)"("DisabledEnum"=w26) -> ()  [unwired: 2 in, 2 out]
    }
  }
  n145 = Obtain Queue(name (unnamed)="Action", element data type="" ("data (can be any type)")) -> (queue out=w3:refnum<queue>)  [unwired: 3 in, 2 out]
  n146 = while {
    tunnel: [w64] -> w4
    tunnel: w3 -> [w63]
    stop <- "Quit" stop-if-true
    # "This loop is a consumer loop."
    n147 = Dequeue Element(queue=w63) -> (queue out=w64:refnum<queue>, element=w65:string)  [unwired: 2 in, 2 out]
    n148 = case shown="\"Idle\", Default" w65 {
      tunnel: w64 -> [w66 _ _ _ w5634 w5935 w6155 _]
      tunnel: w64 -> [_ _ w1795 w3755 _ _ _ _]
      frame "Idle", Default {
        # "0 = SR830_1_ip\n1 = SR830_1_oop\n2 = SR830_2_ip\n3 = SR830_2_oop\n4 = SR830_3_ip\n5 = SR830_3_oop\n6 = SR830_4_ip \n7 = SR830_4_oop \n8 = SR830_5_ip \n9 = SR830_5_oop \n10 = SR830_6_ip \n11 = SR830_6_oop\n12 = SR830_7_ip \n13 = SR830_7_oop\n14 = SR830_8_ip \n15 = SR830_8_oop\n16 = MFLI_V1\n17 = MFLI_I1\n18 = MFLI_V\n19 = MFLI_I\n20= 2400_1_v \n21= 2400_1_i \n22 = 2400_2_v\n23 = 2400_2_i \n24 = 2400_3_v \n25 = 2400_3_i \n26 = 2182A_1_ch1 \n27 = 2182A_1_ch2 \n28 = 2182A_2_ch1 \n29 = 2182A_2_ch2\n30 = 2182A_3_ch1 \n31 = 2182A_3_ch2 \n32 = 2182A_4_ch1 \n33 = 2182A_4_ch2 \n34 = 2636A_smua_v \n35 = 2636A_smua_i \n36 = 2636A_smub_v \n37 = 2636A_smub_i \n38 = time\n39 = iPS_Field\n40 = iPS_Magnet_T\n41 = iPS__SH_T\n42 = iTC _sample_T\n43 = iTC _VTI_T\n44 = iTC _PT1_T\n45 = iTC _PT2_T\n46 = iTC _VTI_P\n47 = 2461_meas_v\n48= 2461_meas_i\n49= Step_Value\n50= HyperLoop_Step\n51= SuperHyper_Step"
        n149 = stacked-sequence {
          tunnel: w66 -> [_ _ _ _ w1791]
          frame #0 {
            # "Read current value of sweep channel"
            # "1 = 2400 1\n2 = 2400 2\n3 = 2400 3\n4 = 2636a smua\n5 = 2636a smub\n6 = do not sweep, just time\n7 =IPS120-10\n8 =2461_smu"
            n150 = property on="sweep" class="RadioBtnsControl (strict)"() -> ("Value"=w68:T6)  [unwired: 2 in, 2 out]
            n151 = case "reads current value from instrument which will be sweeping" shown="\"2400_3\"" w68 {
              tunnel: [w69 w79 w88 w97 w101 0.0 ("Measuremet") w106 w186] -> w67
              frame "2400_1", Default {
                # "reads the voltage on 2400 1"
                n152 = local read "2400 1 addr"() -> (w73:u8)
                n153 = Number To Decimal String(number=w73) -> (decimal integer string=w74:string)  [unwired: 1 in]
                n154 = GPIB Write(0:w74, 1:":READ?") -> (6:w70:errorcluster)  [unwired: 3 in, 1 out]
                n155 = GPIB Read(0:w74, 1:3200, 3:w70) -> (5:w76:string)  [unwired: 2 in, 2 out]
                n156 = String Subset(string=w76, length (rest)=13) -> (substring=w77:string)  [unwired: 1 in]
                n157 = Fract/Exp String To Number(string=w77) -> (number=w69:dbl)  [unwired: 3 in, 1 out]
              }
              frame "2400_2" {
                # "reads the current on 2400 2"
                n158 = local read "2400 2 addr"() -> (w83:u8)
                n159 = Number To Decimal String(number=w83) -> (decimal integer string=w84:string)  [unwired: 1 in]
                n160 = GPIB Write(0:w84, 1:":READ?") -> (6:w80:errorcluster)  [unwired: 3 in, 1 out]
                n161 = GPIB Read(0:w84, 1:3200, 3:w80) -> (5:w86:string)  [unwired: 2 in, 2 out]
                n162 = String Subset(string=w86, offset (0)=14, length (rest)=13) -> (substring=w87:string)
                n163 = Fract/Exp String To Number(string=w87) -> (number=w79:dbl)  [unwired: 3 in, 1 out]
              }
              frame "2400_3" {
                # "reads the voltage on 2400 3"
                n164 = local read "2400 3 addr"() -> (w92:u8)
                n165 = Number To Decimal String(number=w92) -> (decimal integer string=w93:string)  [unwired: 1 in]
                n166 = GPIB Write(0:w93, 1:":READ?") -> (6:w89:errorcluster)  [unwired: 3 in, 1 out]
                n167 = GPIB Read(0:w93, 1:3200, 3:w89) -> (5:w95:string)  [unwired: 2 in, 2 out]
                n168 = String Subset(string=w95, length (rest)=13) -> (substring=w96:string)  [unwired: 1 in]
                n169 = Fract/Exp String To Number(string=w96) -> (number=w88:dbl)  [unwired: 3 in, 1 out]
              }
              frame "2636a_smua" {
                # "reads the voltage on 2636a smua"
                n170 = local read "2336A addr"() -> (w100:refnum<visa-resource-name>)
                n171 = call "SinglePointMeasurement.vi"("Measure"=Measure."Voltage", "Channel"=Channel."a", "VISA resource name 2"=w100) -> ("Measuremet"=w97:dbl)  [unwired: 3 in, 4 out]
              }
              frame "2636a_smub" {
                # "reads the voltage on 2636a smub"
                n172 = local read "2336A addr"() -> (w104:refnum<visa-resource-name>)
                n173 = call "SinglePointMeasurement.vi"("Measure"=Measure."Voltage", "Channel"=Channel."b", "VISA resource name 2"=w104) -> ("Measuremet"=w101:dbl)  [unwired: 3 in, 4 out]
              }
              frame "time_sweep" {
              }
              frame "iPS" {
                n174 = disable-structure shown="Enabled" {
                  disable-tunnel: [w107 w184] -> w106
                  frame Disabled {
                    n175 = stacked-sequence {
                      tunnel: [_ _ _ _ _ _ _ w165 _] -> w107
                      frame #0 {
                        # "initialize interface of HULK SMS"
                        n176 = local read "Hulk_SMS_addr"() -> (w114:refnum<visa-resource-name>)
                        n177 = VISA Open(VISA resource name=w114) -> (VISA resource name=w113:refnum<visa-resource-name>, error out=w112:errorcluster)  [unwired: 4 in]
                        n178 = VISA Clear(VISA resource name=w113, error in (no error)=w112) -> (VISA resource name out=w110:refnum<visa-resource-name>, error out=w109:errorcluster)
                        n179 = property class="Instr"(reference=w110, error in=w109, "General Settings:Timeout Value"=u32 2000) -> (error out=w108:errorcluster)  [unwired: 1 out]
                        n180 = local write item#-1(w108) -> ()
                      }
                      frame #1 {
                        w115 = SMScontrols."UPDATE" ("SMS controls")
                        # "check intialization"
                        n181 = local read "Hulk_SMS_addr"() -> (w119:refnum<visa-resource-name>)
                        n182 = local read item#-1() -> (w118)
                        n183 = call "SMSsendCommand.vi"("HULK SMS address in"=w119, "SMS controls"=w115, "error in"=w118) -> ("HULK SMS address out"=w120:refnum<visa-resource-name>, "error out"=w121:errorcluster)  [unwired: 14 in, 1 out]
                        n184 = call "WaitRS232.vi"("error in"=w121, "delay[160 ms]"=u32 1000) -> ("error out"=w123:errorcluster)  [unwired: 1 in]
                        n185 = call "SMSread.vi"("HULK SMS address in"=w120, "SMS controls"=w115, "error in"=w123) -> ("read buffer"=w116:string, "error out"=w117:errorcluster)  [unwired: 11 in, 4 out]
                        n186 = local write item#-1(w116) -> ()
                        n187 = local write item#-1(w117) -> ()
                      }
                      frame #2 {
                        n188 = Wait (ms)(milliseconds to wait=u32 200) -> ()  [unwired: 1 out]
                      }
                      frame #3 {
                        w125 = SMScontrols."TESLA ON" ("SMS controls")
                        # "set units to tesla"
                        n189 = local read "Hulk_SMS_addr"() -> (w129:refnum<visa-resource-name>)
                        n190 = local read item#-1() -> (w128)
                        n191 = call "SMSsendCommand.vi"("HULK SMS address in"=w129, "SMS controls"=w125, "error in"=w128) -> ("HULK SMS address out"=w130:refnum<visa-resource-name>, "error out"=w131:errorcluster)  [unwired: 14 in, 1 out]
                        n192 = call "WaitRS232.vi"("error in"=w131, "delay[160 ms]"=u32 1000) -> ("error out"=w133:errorcluster)  [unwired: 1 in]
                        n193 = call "SMSread.vi"("HULK SMS address in"=w130, "SMS controls"=w125, "error in"=w133) -> ("read buffer"=w126:string, "error out"=w127:errorcluster)  [unwired: 11 in, 4 out]
                        n194 = local write item#-1(w126) -> ()
                        n195 = local write item#-1(w127) -> ()
                      }
                      frame #4 {
                        w134 = T12."Disabled and Grayed Out" ("Disabled")
                        # "sorry, no control of sweep rate and target\nvalue during sweeping\n\n!!! do not forget to reactivate it in the PAUSE mode!!!"
                      }
                      frame #5 {
                        w138 = SMScontrols."SET RAMP" ("SMS controls")
                        # "preparing HULK SMS!"
                        # "actual sweep rate"
                        # "1sec delay\nbecause HULK is not very bright"
                        # "sets sweep rate for HULK SMS"
                        n196 = local read item#-1() -> (w152)
                        n197 = local read "Hulk_SMS_addr"() -> (w151:refnum<visa-resource-name>)
                        n198 = local read item#-1() -> (w149)
                        n199 = call "SweepRateConversion.vi"("RAMP rate in"=w152, "T/min to A/s (True)"=TRUE) -> ("RAMP rate out"=w150:dbl)
                        n200 = call "SMSsendCommand.vi"("HULK SMS address in"=w151, "SMS controls"=w138, "error in"=w149, "RAMP rate"=w150) -> ("HULK SMS address out"=w145:refnum<visa-resource-name>, "error out"=w146:errorcluster)  [unwired: 13 in, 1 out]
                        n201 = call "WaitRS232.vi"("error in"=w146, "delay[160 ms]"=u32 1000) -> ("error out"=w148:errorcluster)  [unwired: 1 in]
                        n202 = call "SMSread.vi"("HULK SMS address in"=w145, "SMS controls"=w138, "error in"=w148) -> ("read buffer"=w141:string, "error out"=w142:errorcluster)  [unwired: 11 in, 4 out]
                        n203 = Match Pattern(string=w141, regular expression="RAMP RATE:") -> (after substring=w144:string)  [unwired: 1 in, 3 out]
                        n204 = local write item#-1(w141) -> ()
                        n205 = Scan From String(format string="%.f", input string=w144, error in=w142) -> (error out=w139:errorcluster, output 1=w137:dbl)  [unwired: 2 in, 2 out]
                        n206 = local write item#-1(w139) -> ()
                        n207 = call "SweepRateConversion.vi"("RAMP rate in"=w137, "T/min to A/s (True)"=FALSE) -> ("RAMP rate out"=w135:dbl)
                        n208 = local write item#-1(w135) -> ()
                      }
                      frame #6 {
                        w154 = SMScontrols."SET MID" ("SMS controls")
                        # "sets target value for B field sweep"
                        n209 = local read "Hulk_SMS_addr"() -> (w157:refnum<visa-resource-name>)
                        n210 = local read item#-1() -> (w158)
                        n211 = local read item#-1() -> (w156)
                        n212 = call "SMSsendCommand.vi"("HULK SMS address in"=w157, "SMS controls"=w154, "error in"=w158, "MID field value"=w156) -> ("HULK SMS address out"=w162:refnum<visa-resource-name>, "error out"=w160:errorcluster)  [unwired: 13 in, 1 out]
                        n213 = call "WaitRS232.vi"("error in"=w160, "delay[160 ms]"=u32 1000) -> ("error out"=w161:errorcluster)  [unwired: 1 in]
                        n214 = call "SMSread.vi"("HULK SMS address in"=w162, "SMS controls"=w154, "error in"=w161) -> ("read buffer"=w155:string, "error out"=w159:errorcluster)  [unwired: 11 in, 4 out]
                        n215 = local write item#-1(w159) -> ()
                        n216 = local write item#-1(w155) -> ()
                      }
                      frame #7 {
                        # "acquires current output value"
                        n217 = local read "Hulk_SMS_addr"() -> (w168:refnum<visa-resource-name>)
                        n218 = local read item#-1() -> (w167)
                        n219 = call "SMS_GET_OUTPUT.vi"("CRYogenic:("=w167, "Hulk_SMS_addr"=w168) -> ("error IO"=w164:errorcluster, "read buffer"=w166:string, "Numeric"=w165:dbl)
                        n220 = local write item#-1(w164) -> ()
                        n221 = local write item#-1(w166) -> ()
                      }
                      frame #8 {
                        # "activates ramping"
                        n222 = local read item#-1() -> (w176)
                        n223 = Equal?(x=w176, y=0.0) -> (x = y?=w174:bool)
                        n224 = Select(t=SMScontrols."RAMP ZERO" ("SMS controls"), s=w174, f=SMScontrols."RAMP MID" ("SMS controls")) -> (s? t:f=w171:T14)
                        n225 = local read "Hulk_SMS_addr"() -> (w178:refnum<visa-resource-name>)
                        n226 = local read item#-1() -> (w177)
                        n227 = call "SMSsendCommand.vi"("HULK SMS address in"=w178, "SMS controls"=w171, "error in"=w177) -> ("HULK SMS address out"=w181:refnum<visa-resource-name>, "error out"=w180:errorcluster)  [unwired: 14 in, 1 out]
                        n228 = call "WaitRS232.vi"("error in"=w180, "delay[160 ms]"=u32 1000) -> ("error out"=w182:errorcluster)  [unwired: 1 in]
                        n229 = call "SMSread.vi"("HULK SMS address in"=w181, "SMS controls"=w171, "error in"=w182) -> ("read buffer"=w169:string, "error out"=w170:errorcluster)  [unwired: 11 in, 4 out]
                        n230 = local write item#-1(w170) -> ()
                        n231 = local write item#-1(w169) -> ()
                      }
                    }
                  }
                  frame Enabled {
                    # "preparing Teslatron_iPS_Field"
                    # "Measure magnetic field on Teslatron_iPS_Field"
                    n232 = property on="iPS_addr_sweep" class="VISAName"() -> ("Value"=w185:refnum<visa-resource-name>)  [unwired: 2 in, 2 out]
                    n233 = call "iPSread.vi"("iPSreadCtrl"=iPSreadCtrl."OutputField", "VISA resource name"=w185) -> ("number"=w184:dbl)  [unwired: 6 in, 3 out]
                  }
                }
              }
              frame "iTC" {
                n234 = disable-structure shown="Enabled" {
                  disable-tunnel: [w194 w198] -> w186
                  frame Disabled {
                    w197 = u16 0 items=["Volts", "Current", "Auto Resistance", "Manual Resistance", "Digitize Voltage", "Digitize Current"] ("Function (0: Volts)")
                    w191 = u16 1 items=["Volts", "Current"] ("Function (0: Volts)")
                    n235 = property on="iTC_addr_sweep" class="VISAName"() -> ("Value"=w193:refnum<visa-resource-name>)  [unwired: 2 in, 2 out]
                    n236 = call <instrlib>:"Configure Source Limit Level.vi"("Source Limit (1.0)"=5.0, "Function (0: Volts)"=w191, "VISA resource name"=w193) -> ("error out"=w189:errorcluster, "VISA resource name out"=w192:refnum<visa-resource-name>)  [unwired: 7 in]
                    n237 = call <instrlib>:"Configure Measurement Function.vi"("error in (no error)"=w189, "Function (0: Volts)"=w197, "VISA resource name"=w192) -> ("error out"=w188:errorcluster, "VISA resource name out"=w196:refnum<visa-resource-name>)  [unwired: 7 in]
                    n238 = call <instrlib>:"Enable Output.vi"("error in (no error)"=w188, "VISA resource name"=w196) -> ("error out"=w187:errorcluster, "VISA resource name out"=w195:refnum<visa-resource-name>)  [unwired: 8 in]
                    n239 = call <instrlib>:"Get Source Level.vi"("error in (no error)"=w187, "VISA resource name"=w195) -> ("Current Level Out"=w194:dbl)  [unwired: 6 in, 3 out]
                  }
                  frame Enabled {
                    n240 = property on="iTC_addr_sweep" class="VISAName"() -> ("Value"=w200:refnum<visa-resource-name>)  [unwired: 2 in, 2 out]
                    n241 = call "iTCread.vi"("VISA resource name"=w200, "iTCreadCtrl"=iTCreadCtrl."Sample Temp") -> ("number"=w198:dbl)  [unwired: 5 in, 3 out]
                  }
                }
              }
            }
            n242 = property on="Sweep Channel" class="DigNum (strict)"("Value"=w67) -> ()  [unwired: 2 in, 2 out]
          }
          frame #1 {
            # "Read Current value of step channel"
            n243 = property on="Step Loop" class="Bool (strict)"() -> ("Value"=w201:bool)  [unwired: 2 in, 2 out]
            n244 = case shown="True" w201 {
              frame False {
                w202 = 9999999.0 ("Step Channel")
                n245 = property on="Step Channel" class="DigNum (strict)"("Value"=w202) -> ()  [unwired: 2 in, 2 out]
                n246 = property on="Hyper Channel" class="DigNum (strict)"("Value"=w202) -> ()  [unwired: 2 in, 2 out]
              }
              frame True {
                # "1 = 2400 1\n2 = 2400 2\n3 = 2400 3\n4 = 2636a smua\n5 = 2636a smub\n6 = do not sweep, just time\n7 =IPS120-10\n8 =2461_smu"
                n247 = property on="step" class="RadioBtnsControl (strict)"() -> ("Value"=w204:T8)  [unwired: 2 in, 2 out]
                n248 = case "reads current value from instrument which will be sweeping" shown="\"2461_Curr\"" w204 {
                  tunnel: [w206 w216 w225 w229 0.0 ("Measuremet") w235 w236 w239] -> w203
                  frame "V2400_1_Step", Default {
                    # "reads the voltage on 2400 1"
                    n249 = property on="2400_1_addr_step" class="DigNum (strict)"() -> ("Value"=w205:u8)  [unwired: 2 in, 2 out]
                    n250 = Number To Decimal String(number=w205) -> (decimal integer string=w210:string)  [unwired: 1 in]
                    n251 = GPIB Write(0:w210, 1:":READ?") -> (6:w207:errorcluster)  [unwired: 3 in, 1 out]
                    n252 = GPIB Read(0:w210, 1:3200, 3:w207) -> (5:w212:string)  [unwired: 2 in, 2 out]
                    n253 = String Subset(string=w212, length (rest)=13) -> (substring=w213:string)  [unwired: 1 in]
                    n254 = Fract/Exp String To Number(string=w213) -> (number=w206:dbl)  [unwired: 3 in, 1 out]
                  }
                  frame "V2400_2_step" {
                    # "reads the current on 2400 2"
                    n255 = property on="2400_2_addr_step" class="DigNum (strict)"() -> ("Value"=w214:u8)  [unwired: 2 in, 2 out]
                    n256 = Number To Decimal String(number=w214) -> (decimal integer string=w220:string)  [unwired: 1 in]
                    n257 = GPIB Write(0:w220, 1:":READ?") -> (6:w217:errorcluster)  [unwired: 3 in, 1 out]
                    n258 = GPIB Read(0:w220, 1:3200, 3:w217) -> (5:w222:string)  [unwired: 2 in, 2 out]
                    n259 = String Subset(string=w222, offset (0)=14, length (rest)=13) -> (substring=w223:string)
                    n260 = Fract/Exp String To Number(string=w223) -> (number=w216:dbl)  [unwired: 3 in, 1 out]
                  }
                  frame "2636_smua_step" {
                    # "reads the voltage on 2636a smua"
                    n261 = property on="2336A_addr_step" class="VISAName"() -> ("Value"=w224:refnum<visa-resource-name>)  [unwired: 2 in, 2 out]
                    n262 = call "SinglePointMeasurement.vi"("Measure"=Measure."Voltage", "Channel"=Channel."a", "VISA resource name 2"=w224) -> ("Measuremet"=w225:dbl)  [unwired: 3 in, 4 out]
                  }
                  frame "2636_smub_step" {
                    # "reads the voltage on 2636a smub"
                    n263 = property on="2336A_addr_step" class="VISAName"() -> ("Value"=w228:refnum<visa-resource-name>)  [unwired: 2 in, 2 out]
                    n264 = call "SinglePointMeasurement.vi"("Measure"=Measure."Voltage", "Channel"=Channel."b", "VISA resource name 2"=w228) -> ("Measuremet"=w229:dbl)  [unwired: 3 in, 4 out]
                  }
                  frame "time_step" {
                  }
                  frame "iPS_step" {
                    # "Measure magnetic field on IPS"
                    n265 = property on="iPS _addr_step" class="VISAName"() -> ("Value"=w234:refnum<visa-resource-name>)  [unwired: 2 in, 2 out]
                    n266 = call "iPSread.vi"("iPSreadCtrl"=iPSreadCtrl."OutputField", "VISA resource name"=w234) -> ("number"=w235:dbl)  [unwired: 6 in, 3 out]
                  }
                  frame "iTC_step" {
                    n267 = property on="iTC_addr_step" class="VISAName"() -> ("Value"=w238:refnum<visa-resource-name>)  [unwired: 2 in, 2 out]
                    n268 = call "iTCread.vi"("VISA resource name"=w238, "iTCreadCtrl"=iTCreadCtrl."Sample Temp") -> ("number"=w236:dbl)  [unwired: 5 in, 3 out]
                  }
                  frame "2461_Curr" {
                    n269 = property on="2461_addr_sweep" class="VISAName"() -> ("Value"=w240:refnum<visa-resource-name>)  [unwired: 2 in, 2 out]
                    n270 = call <instrlib>:"Get Source Level.vi"("VISA resource name"=w240) -> ("Current Level Out"=w239:dbl)  [unwired: 7 in, 3 out]
                  }
                }
                n271 = property on="Step Channel" class="DigNum (strict)"("Value"=w203) -> ()  [unwired: 2 in, 2 out]
              }
            }
          }
          frame #2 {
            # "Read Current value of hyp[er loop channel"
            n272 = property on="HyperLoop" class="Bool (strict)"() -> ("Value"=w241:bool)  [unwired: 2 in, 2 out]
            n273 = case shown="True" w241 {
              frame False {
                n274 = property on="Hyper Channel" class="DigNum (strict)"("Value"=9999999.0 ("Step Channel")) -> ()  [unwired: 2 in, 2 out]
              }
              frame True {
                # "1 = 2400 1\n2 = 2400 2\n3 = 2400 3\n4 = 2636a smua\n5 = 2636a smub\n6 = do not sweep, just time\n7 =IPS120-10\n8 =2461_smu"
                n275 = property on="step_hyper" class="RadioBtnsControl (strict)"() -> ("Value"=w244:T9)  [unwired: 2 in, 2 out]
                n276 = case "reads current value from instrument which will be sweeping" shown="\"iTC_HyperLoop\"" w244 {
                  tunnel: [w246 w256 w265 w269 0.0 ("Measuremet") w275 w277] -> w243
                  frame "2400_1_HyperLoop", Default {
                    # "reads the voltage on 2400 1"
                    n277 = property on="2400_1_addr_hyper" class="DigNum (strict)"() -> ("Value"=w245:u8)  [unwired: 2 in, 2 out]
                    n278 = Number To Decimal String(number=w245) -> (decimal integer string=w250:string)  [unwired: 1 in]
                    n279 = GPIB Write(0:w250, 1:":READ?") -> (6:w247:errorcluster)  [unwired: 3 in, 1 out]
                    n280 = GPIB Read(0:w250, 1:3200, 3:w247) -> (5:w252:string)  [unwired: 2 in, 2 out]
                    n281 = String Subset(string=w252, length (rest)=13) -> (substring=w253:string)  [unwired: 1 in]
                    n282 = Fract/Exp String To Number(string=w253) -> (number=w246:dbl)  [unwired: 3 in, 1 out]
                  }
                  frame "2400_2_HyperLoop" {
                    # "reads the current on 2400 2"
                    n283 = property on="2400_2_addr_hyper" class="DigNum (strict)"() -> ("Value"=w254:u8)  [unwired: 2 in, 2 out]
                    n284 = Number To Decimal String(number=w254) -> (decimal integer string=w260:string)  [unwired: 1 in]
                    n285 = GPIB Write(0:w260, 1:":READ?") -> (6:w257:errorcluster)  [unwired: 3 in, 1 out]
                    n286 = GPIB Read(0:w260, 1:3200, 3:w257) -> (5:w262:string)  [unwired: 2 in, 2 out]
                    n287 = String Subset(string=w262, offset (0)=14, length (rest)=13) -> (substring=w263:string)
                    n288 = Fract/Exp String To Number(string=w263) -> (number=w256:dbl)  [unwired: 3 in, 1 out]
                  }
                  frame "2636_smua_HyperLoop" {
                    # "reads the voltage on 2636a smua"
                    n289 = property on="2336A_addr_hyper" class="VISAName"() -> ("Value"=w264:refnum<visa-resource-name>)  [unwired: 2 in, 2 out]
                    n290 = call "SinglePointMeasurement.vi"("Measure"=Measure."Voltage", "Channel"=Channel."a", "VISA resource name 2"=w264) -> ("Measuremet"=w265:dbl)  [unwired: 3 in, 4 out]
                  }
                  frame "2636_smub_HyperLoop" {
                    # "reads the voltage on 2636a smub"
                    n291 = property on="2336A_addr_hyper" class="VISAName"() -> ("Value"=w268:refnum<visa-resource-name>)  [unwired: 2 in, 2 out]
                    n292 = call "SinglePointMeasurement.vi"("Measure"=Measure."Voltage", "Channel"=Channel."b", "VISA resource name 2"=w268) -> ("Measuremet"=w269:dbl)  [unwired: 3 in, 4 out]
                  }
                  frame "time_HyperLoop" {
                  }
                  frame "iPS_HyperLoop" {
                    # "Measure magnetic field on IPS"
                    n293 = property on="iPS _addr_hyper" class="VISAName"() -> ("Value"=w273:refnum<visa-resource-name>)  [unwired: 2 in, 2 out]
                    n294 = call "iPSread.vi"("iPSreadCtrl"=iPSreadCtrl."OutputField", "VISA resource name"=w273) -> ("number"=w275:dbl)  [unwired: 6 in, 3 out]
                  }
                  frame "iTC_HyperLoop" {
                    n295 = property on="iTC_addr_hyper" class="VISAName"() -> ("Value"=w276:refnum<visa-resource-name>)  [unwired: 2 in, 2 out]
                    n296 = call "iTCread.vi"("VISA resource name"=w276, "iTCreadCtrl"=iTCreadCtrl."Sample Temp") -> ("number"=w277:dbl)  [unwired: 5 in, 3 out]
                  }
                }
